vi "CRYReport Global.vi"() -> ()   [LabVIEW 2013]
uses:
  CRYWindow/DataView/Control/CRYDrag Graph.ctl
panel:
  in  "pathTemplate":path
  in  "bCallback":bool
  in  "bReportSaved":bool
  in  "bReportOpend":bool
  in  "ctrlTXButtonBar":refnum<k7>
  in  "cDropData":T1
  in  "sPageInfo":string
  in  "cPrintPage":T2
  in  "nIDFActiveXEdit":i16
  in  "cBootReport":T3
  in  "ctlTXTextControl":refnum<k7>
  in  "pathActiveX":path
  in  "pathTemp":path
  in  "cBootFrame":T3
  in  "cFrameList":T4
  in  "cBootVIEW":T3
  in  "cFrame":T5
  in  "pathReportLog":path
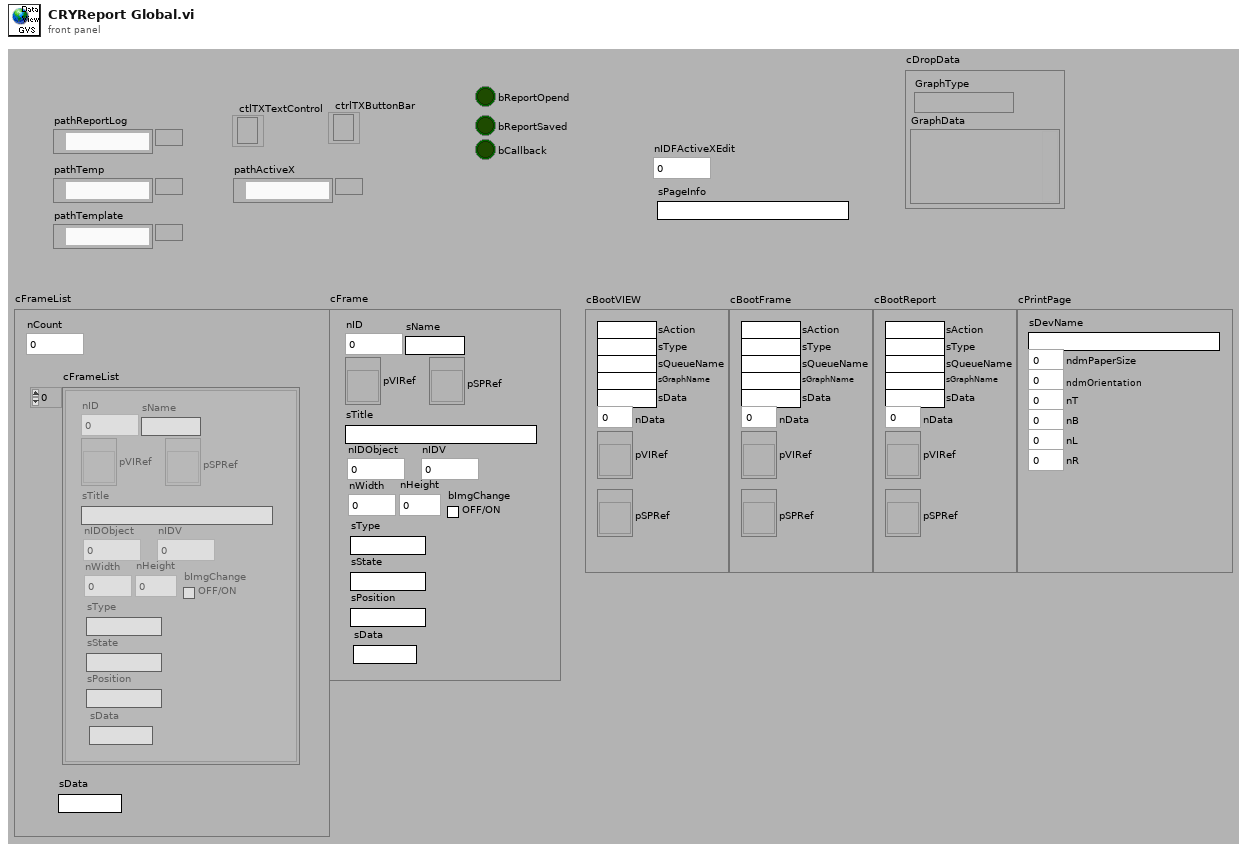
[diagram p1: front panel]
types:
  T1 = typedef "CRYDrag Graph.ctl" = cluster{"GraphType":string, "GraphData":variant}
  T2 = cluster{"sDevName":string, "ndmPaperSize":i32, "ndmOrientation":i32, "nT":i32, "nB":i32, "nL":i32, "nR":i32}
  T3 = cluster{"sAction":string, "sType":string, "sQueueName":string, "sGraphName":string, "sData":string, "nData":i32, "pVIRef":refnum<vi>, "pSPRef":refnum<vi>}
  T4 = cluster{"nCount":i16, "cFrameList":cluster{"nID":i16, "sName":string, "pVIRef":refnum<vi>, "pSPRef":refnum<vi>, "sTitle":string, "nIDObject":i16, "nIDV":i16, "nWidth":i16, "nHeight":i16, "bImgChange":bool, "sType":string, "sState":string, "sPosition":string, "sData":string}[], "sData":string}
  T5 = cluster{"nID":i16, "sName":string, "pVIRef":refnum<vi>, "pSPRef":refnum<vi>, "sTitle":string, "nIDObject":i16, "nIDV":i16, "nWidth":i16, "nHeight":i16, "bImgChange":bool, "sType":string, "sState":string, "sPosition":string, "sData":string}
diagram:
